vi "Destroy Raw Data Queue.vi"(8 "error in (no error)":errorcluster) -> (0 "error out":errorcluster)   [LabVIEW 2017]
uses:
  Application Control/Application Globals.vi
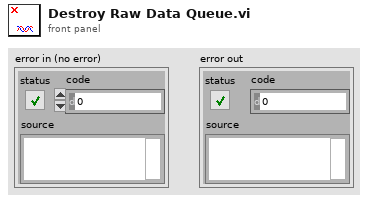
[diagram p1: front panel]
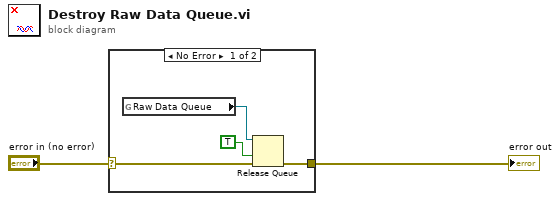
[diagram p0: block diagram]
diagram:
  n1 = case shown="No Error" "error in (no error)" {
    selector: "error in (no error)" -> [w3 w7]
    tunnel: [w4 w7] -> w1
    frame No Error {
      n2 = global read "Application Globals.vi" "Raw Data Queue"() -> (w5:refnum<queue>)
      n3 = Release Queue(queue=w5, force destroy? (F)=TRUE, error in (no error)=w3) -> (error out=w4:errorcluster)  [unwired: 2 out]
    }
    frame Error {
    }
  }
  "error out" <- w1
